vi "常规五参数测量数据区.vi"(11 "数组":u16[](array[numeric]) format="%04xH") -> (3 "测量数据区":T1)   [LabVIEW 2016, in "斯坦道原位多参数.lvlib"]
panel:
  # "共占用30 WORD"
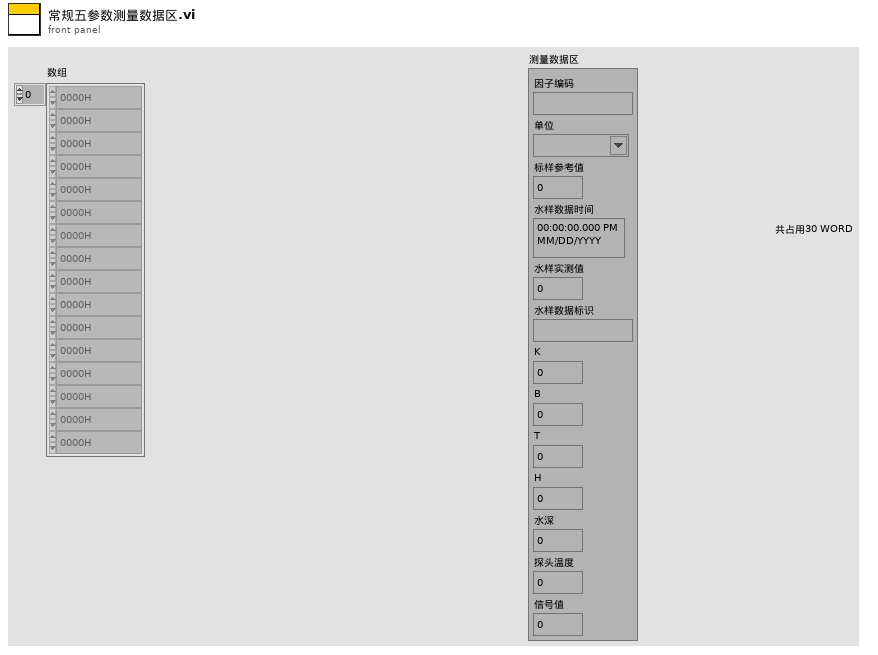
[diagram p1: front panel]
types:
  T1 = cluster{"因子编码":string, "单位":string, "标样参考值":sgl, "水样数据时间":timestamp, "水样实测值":sgl, "水样数据标识":string, "K":sgl, "B":sgl, "T":sgl, "H":sgl, "水深":sgl, "探头温度":sgl, "信号值":sgl}
  T2 = cluster{string, string, "FLOAT":sgl, "time stamp":timestamp, "数值":sgl, "string":string, "FLOAT":sgl, "FLOAT":sgl, "FLOAT":sgl, "FLOAT":sgl, "FLOAT":sgl, "FLOAT":sgl, "FLOAT":sgl}
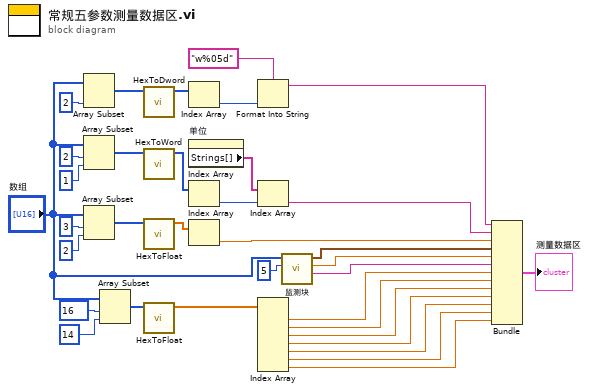
[diagram p0: block diagram]
diagram:
  n1 = Array Subset(array="数组", length=2 ("长度")) -> (w35:u16[])  [unwired: 1 in]
  n2 = Array Subset(array="数组", index=2 ("索引"), length=1 ("长度")) -> (w30:u16[])
  n3 = Array Subset(array="数组", index=3 ("索引"), length=2 ("长度")) -> (w26:u16[])
  n4 = Array Subset(array="数组", index=16 ("索引"), length=14 ("长度")) -> (w16:u16[])
  n5 = call "HexToDword.vi"("数组"=w35) -> ("DWORD"=w33:i32[])  [unwired: 10 in]
  n6 = call "HexToWord.vi"("数组"=w30) -> ("WORD"=w29:u16[])  [unwired: 10 in]
  n7 = call "HexToFloat.vi"("数组"=w26) -> ("FLOAT"=w25:sgl[])  [unwired: 10 in]
  n8 = call "HexToFloat.vi"("数组"=w16) -> ("FLOAT"=w15:sgl[])  [unwired: 10 in]
  n9 = Index Array(array=w33) -> (element=w4:i32)  [unwired: 1 in]
  n10 = property on="单位" class="CmbBox"() -> ("Strings[]"=w6:string[])  [unwired: 2 in, 2 out]
  n11 = Index Array(array=w29) -> (element=w8:u16)  [unwired: 1 in]
  n12 = Index Array(array=w25) -> (element=w24:sgl)  [unwired: 1 in]
  n13 = Format Into String(format string="w%05d" ("格式字符串"), w4) -> (resulting string=w3:string)  [unwired: 2 in, 1 out]
  n14 = Index Array(array=w6, index=w8) -> (element=w7:string)
  n15 = Index Array(array=w15) -> (element #1=w14:sgl, element #2=w13:sgl, element #3=w12:sgl, element #4=w11:sgl, element #5=w10:sgl, element #6=w2:sgl, element #7=w1:sgl)  [unwired: 7 in]
  n16 = call "监测块.vi"("索引"=5, "数组"="数组") -> ("string"=w21:string, "数值"=w22:sgl, "time stamp"=w23:timestamp)  [unwired: 7 in]
  n17 = Bundle(w3, w7, "FLOAT"=w24, "time stamp"=w23, "数值"=w22, "string"=w21, "FLOAT"=w14, "FLOAT"=w13, "FLOAT"=w12, "FLOAT"=w11, "FLOAT"=w10, "FLOAT"=w2, "FLOAT"=w1) -> (→"测量数据区":T2)  [unwired: 1 in]
